vi "Pressure Ranges.vi"() -> (0 "Pressure Ranges":dbl[unit][](array[numeric])=[0.1333, 1.333, 13.33, 133.3, 133.3, 1333.0, 13330.0, 133300.0, 133300.0, 1333000.0, 13330000.0, 0.1, 1.0, 10.0, 100.0, 100.0, 1000.0, 10000.0, 100000.0, 100000.0, 1000000.0, 10000000.0, 1.0, 10.0, 100.0, 1000.0, 10000.0, 100000.0, 1000000.0])   [LabVIEW 2011, in "MGC647C.lvlib"]
doc: "This VI provides full scale pressure ranges supported by the instrument."
uses:
  <instrlib>/MGC647C/MGC647C.lvlib
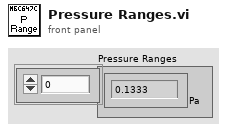
[diagram p1: front panel]
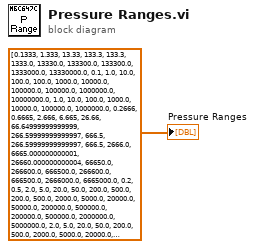
[diagram p0: block diagram]
diagram:
  "Pressure Ranges" <- dbl[unit][] [0.1333, 1.333, 13.33, 133.3, 133.3, 1333.0, 13330.0, 133300.0, 133300.0, 1333000.0, 13330000.0, 0.1, 1.0, 10.0, 100.0, 100.0, 1000.0, 10000.0, 100000.0, 100000.0, 1000000.0, 10000000.0, 1.0, 10.0, 100.0, 1000.0, 10000.0, 100000.0, 1000000.0, 0.2666, 0.6665, 2.666, 6.665, 26.66, 66.64999999999999, 266.59999999999997, 666.5, 266.59999999999997, 666.5, 2666.0, 6665.000000000001, 26660.000000000004, 66650.0, 266600.0, 666500.0, 266600.0, 666500.0, 2666000.0, 6665000.0, 0.2, 0.5, 2.0, 5.0, 20.0, 50.0, 200.0, 500.0, 200.0, 500.0, 2000.0, 5000.0, 20000.0, 50000.0, 200000.0, 500000.0, 200000.0, 500000.0, 2000000.0, 5000000.0, 2.0, 5.0, 20.0, 50.0, 200.0, 500.0, 2000.0, 5000.0, 20000.0, 50000.0, 200000.0, 500000.0, 2000000.0, 5000000.0, 1000000.0, 2000000.0, 5000000.0, 10000000.0] ("array")
